vi "SetFocusToUI.vi"(8 "error in (no error)":errorcluster, 11 "Flex  Dialog (Actor) in":refnum<class "Flex Dialog (Actor).lvclass">) -> (0 "error out":errorcluster, 3 "Flex  Dialog (Actor) out":refnum<class "Flex Dialog (Actor).lvclass">)   [LabVIEW 2014, in "Flex UI Dialog (Actor).lvlib" / "Flex Dialog (Actor).lvclass"]
uses:
  Flex Dialog (Actor).lvclass
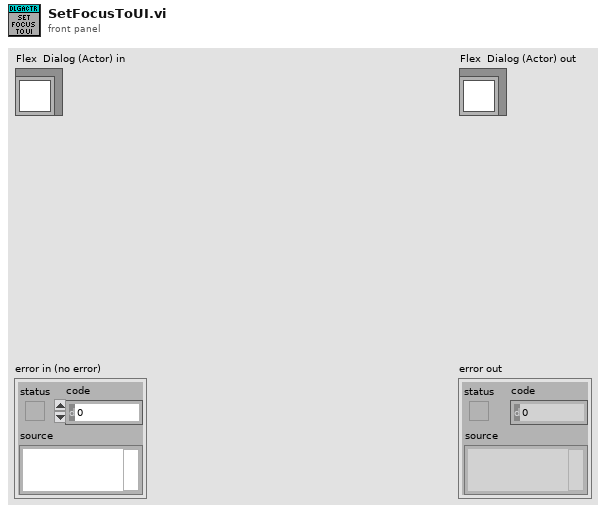
[diagram p1: front panel]
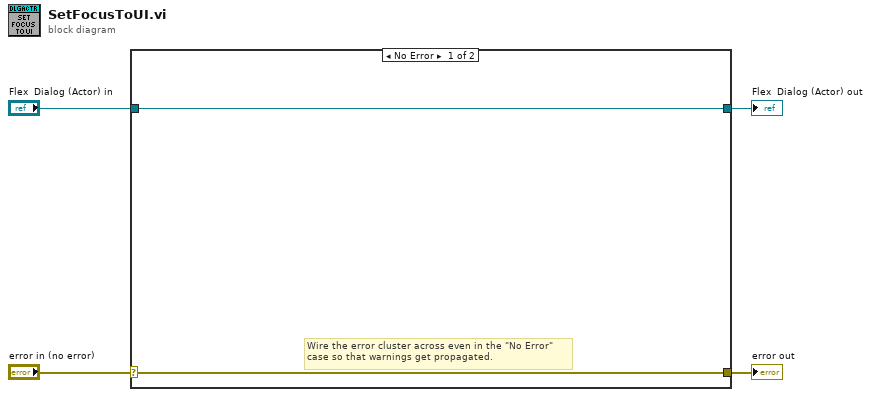
[diagram p0: block diagram]
diagram:
  n1 = case shown="No Error" "error in (no error)" {
    selector: "error in (no error)" -> [w5 w8]
    tunnel: [w5 w8] -> w3
    tunnel: [w6 w7] -> w1
    tunnel: "Flex  Dialog (Actor) in" -> [w6 w7]
    frame No Error {
      # "Wire the error cluster across even in the \"No Error\"\ncase so that warnings get propagated."
    }
    frame Error {
    }
  }
  "error out" <- w3
  "Flex  Dialog (Actor) out" <- w1
